vi "Send Launch Job and Wait for Reply.vi"(8 "error in (no error)":errorcluster, 9 "JSON":string, 10 "Job":refnum<class "Job.lvclass">, 11 "Web Request in":refnum<class "Web Request.lvclass">) -> (0 "error out":errorcluster, 2 "Result String":string)   [LabVIEW 2014]
uses:
  Classes/Job/Job.lvclass
  <vilib>/wsapi/Web Request.lvclass
  Controls/Job Results - STYP.ctl
  Actors/CI Mediator/CI Mediator Messages/Launch Job Msg/Launch Job Msg.lvclass/Launch Job Msg.ctl
  <vilib>/ActorFramework/Message Enqueuer/Message Enqueuer.lvclass/Message Enqueuer.ctl
  <vilib>/ActorFramework/Message Enqueuer/Enqueue.vi
  <vilib>/ActorFramework/Message Priority Queue/Priority Enqueue.vi
  Actors/CI Mediator/CI Mediator Messages/Launch Job Msg/Launch Job Msg.lvclass
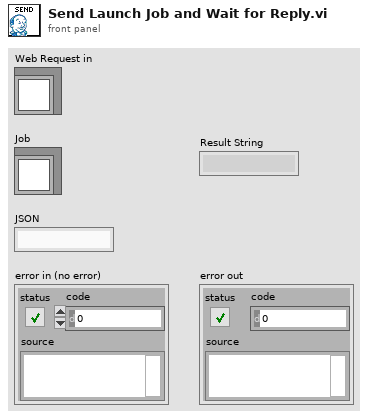
[diagram p1: front panel]
types:
  T1 = typedef "Job Results - STYP.ctl" = cluster{"Status":u16, "Text":string, "Executor Number":i32}
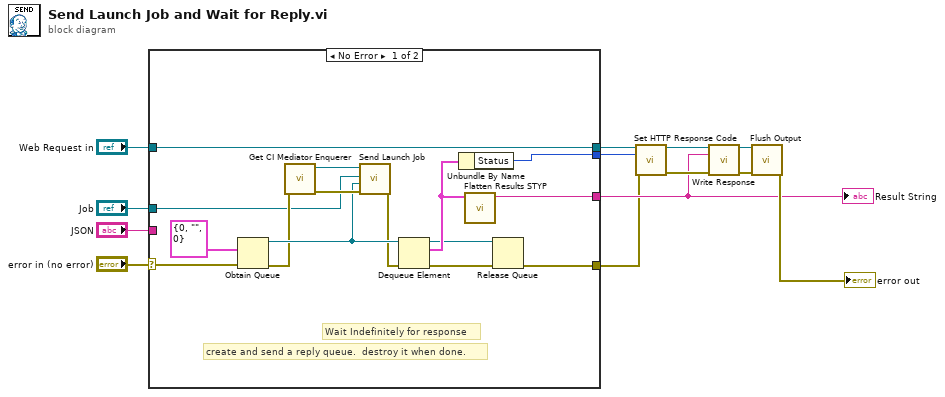
[diagram p0: block diagram]
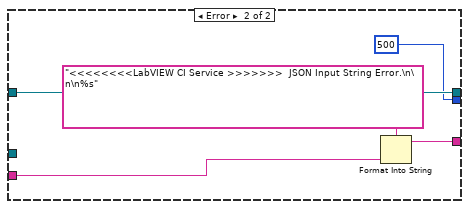
[diagram p2: hidden frame]
diagram:
  n1 = case shown="No Error" "error in (no error)" {
    selector: "error in (no error)" -> [w22 _]
    tunnel: [w26 w30] -> w2
    tunnel: [w15 _] -> w1
    tunnel: [w16 u16 500 ("Status")] -> w3
    tunnel: [w27 w33] -> w5
    tunnel: "Web Request in" -> [w27 w33]
    tunnel: "JSON" -> [_ w29]
    tunnel: "Job" -> [w18 _]
    frame No Error {
      # "create and send a reply queue.  destroy it when done."
      # "Wait Indefinitely for response"
      n2 = Obtain Queue(element data type=T1 {"Status"=0, "Text"="", "Executor Number"=0} ("element"), error in (no error)=w22) -> (queue out=w21:refnum<queue>, error out=w20:errorcluster)  [unwired: 3 in, 1 out]
      n3 = call "Get CI Mediator Enquerer.vi"("error in (no error)"=w20) -> ("error out"=w23:errorcluster, "Enquerer"=w25:refnum<class "Message Enqueuer.lvclass">)  [unwired: 9 in]
      n4 = call "Send Launch Job.vi"("error in (no error)"=w23, "Reply Queue"=w21, "Job.lvclass"=w18, "Message Enqueuer"=w25) -> ("error out"=w19:errorcluster)  [unwired: 6 in, 1 out]
      n5 = Dequeue Element(queue=w21, error in (no error)=w19) -> (queue out=w14:refnum<queue>, element=w17:T1, error out=w28:errorcluster)  [unwired: 1 in, 1 out]
      n6 = Unbundle By Name(w17) -> ("Status"=w16:u16)
      n7 = call "Flatten Results STYP.vi"("Results"=w17) -> ("Result String"=w26:string)  [unwired: 10 in]
      n8 = Release Queue(queue=w14, error in (no error)=w28) -> (error out=w15:errorcluster)  [unwired: 1 in, 2 out]
    }
    frame Error {
      n9 = Format Into String(format string="<<<<<<<<LabVIEW CI Service >>>>>>>  JSON Input String Error.\n\n\n%s" ("Text"), w29) -> (resulting string=w30:string)  [unwired: 2 in, 1 out]
    }
  }
  "Result String" <- w2
  n10 = call <vilib>:"Set HTTP Response Code.vi"("LabVIEW Web Service Request"=w5, "response code (200)"=w3, "error in (no error)"=w1) -> ("LabVIEW Web Service Request out"=w6:refnum<class "Web Request.lvclass">, "error out"=w7:errorcluster)  [unwired: 11 in]
  n11 = call <vilib>:"Write Response.vi"("LabVIEW Web Service Request"=w6, "response string"=w2, "error in (no error)"=w7) -> ("LabVIEW Web Service Request out"=w9:refnum<class "Web Request.lvclass">, "error out"=w8:errorcluster)  [unwired: 11 in]
  n12 = call <vilib>:"Flush Output.vi"("LabVIEW Web Service Request"=w9, "error in (no error)"=w8) -> ("error out"=→"error out":errorcluster)  [unwired: 12 in, 1 out]
